vi "Parse Data Channel Property.vi"(8 "error in (no error)":errorcluster, 11 "Item Informations array":T1[](array[typedef])) -> (0 "error out":errorcluster, 3 "Item Informations array(parsed)":T1[](array[typedef]))   [LabVIEW 2023, in "Vires VTD System Explorer.lvlib"]
uses:
  Vires VTD System Explorer.lvlib
  Item Informations.ctl
  <vilib>/NI VeriStand/Custom Device API/Custom Device Item Info.ctl
  <vilib>/NI VeriStand/Custom Device API/Custom Device Channel.ctl
  <vilib>/NI VeriStand/Custom Device API/Custom Device Channel Type.ctl
  Data Channel Custom Property.ctl
  <vilib>/NI VeriStand/Custom Device API/Custom Device API.lvlib
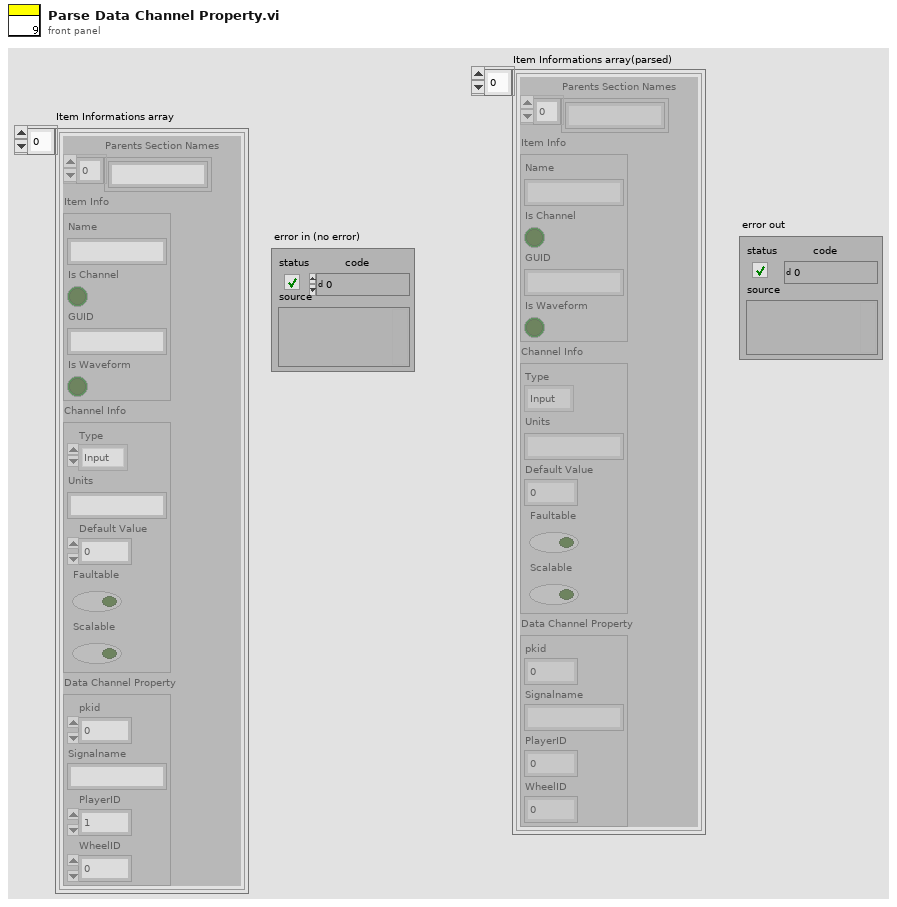
[diagram p1: front panel]
types:
  T1 = typedef "Vires VTD System Explorer.lvlib/Item Informations.ctl" = cluster{"Parents Section Names":string[], "Item Info":T2, "Channel Info":T3, "Data Channel Property":T5}
  T2 = typedef "Custom Device API.lvlib/Custom Device Item Info.ctl" = cluster{"Name":string, "Is Channel":bool, "GUID":string, "Is Waveform":bool}
  T3 = typedef "Custom Device API.lvlib/Custom Device Channel.ctl" = cluster{"Type":T4, "Units":string, "Default Value":dbl, "Faultable":bool, "Scalable":bool}
  T4 = typedef "Custom Device API.lvlib/Custom Device Channel Type.ctl" = enum16{"Input", "Output"}
  T5 = typedef "Vires VTD System Explorer.lvlib/Data Channel Custom Property.ctl" = cluster{"pkid":u32, "Signalname":string, "PlayerID":u8, "WheelID":i32}
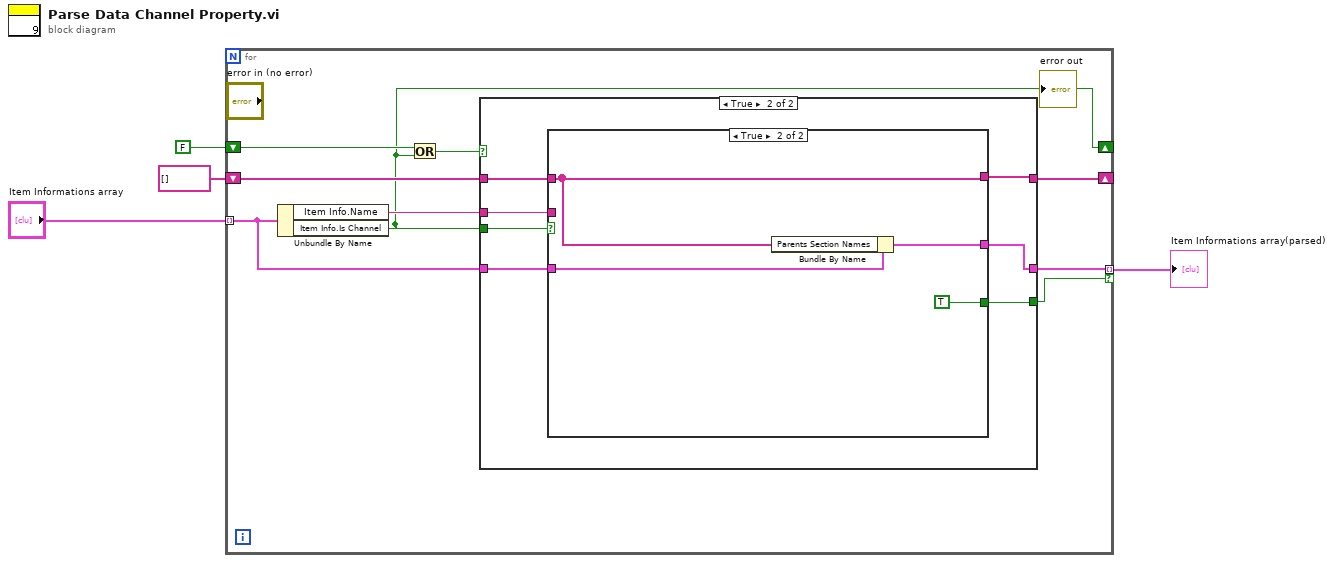
[diagram p0: block diagram]
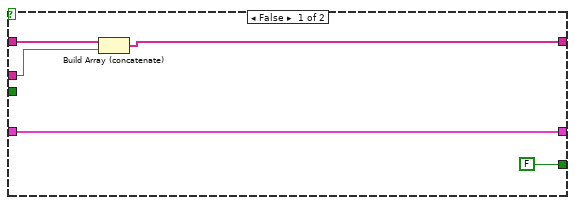
[diagram p2: hidden frame]
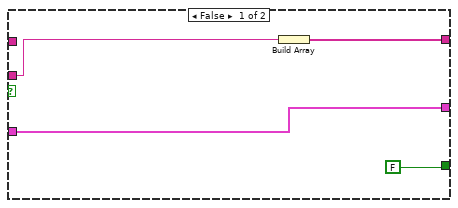
[diagram p3: hidden frame]
diagram:
  n1 = for {
    tunnel: "Item Informations array" -> [w8] mode=indexing
    shift-right: [w5] -> _
    shift-left: FALSE -> [w13]
    shift-right: [w9] -> _
    shift-left: string[] [] -> [w10]
    tunnel: [w7] -> w1 mode=indexing if=w6
    n2 = Unbundle By Name(w8) -> ("Item Info.Name"=w11:string, "Item Info.Is Channel"=w5:bool)
    n3 = Or(x=w13, y=w5) -> (x .or. y?=w12:bool)
    n4 = case shown="True" w12 {
      tunnel: w11 -> [w17 w20]
      tunnel: w10 -> [w18 w24]
      tunnel: [w16 w19] -> w9
      tunnel: w8 -> [w15 w23]
      tunnel: [w15 w22] -> w7
      tunnel: [FALSE w21] -> w6
      tunnel: w5 -> [_ w25]
      frame False {
        n5 = Build Array (concatenate)(w18, w17) -> (w16:string[])
      }
      frame True {
        n6 = case shown="True" w25 {
          tunnel: w24 -> [_ w30]
          tunnel: w23 -> [w28 w33]
          tunnel: [w28 w32] -> w22
          tunnel: [FALSE TRUE] -> w21
          tunnel: w20 -> [w27 _]
          tunnel: [w26 w30] -> w19
          frame False {
            n7 = Build Array(w27) -> (w26:string[])
          }
          frame True {
            n8 = Bundle By Name(cluster=w33, "Parents Section Names"=w30) -> (w32:T1)
          }
        }
      }
    }
  }
  "Item Informations array(parsed)" <- w1
